vi "tabelUmrechnung.vi"(9 "Tabel Positon":dbl, 10 "Inspect":bool) -> (2 "In Range?":bool, 3 "Numerisch":dbl)   [LabVIEW 2020]
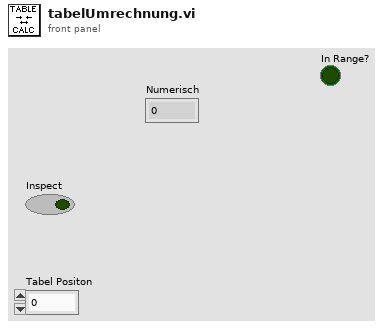
[diagram p1: front panel]
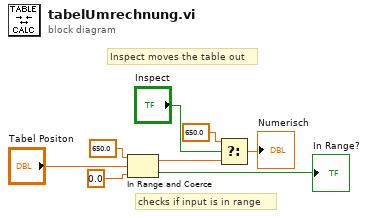
[diagram p0: block diagram]
diagram:
  # "checks if input is in range"
  # "Inspect moves the table out"
  n1 = In Range and Coerce(upper limit=650.0 ("Obergrenze"), x="Tabel Positon", lower limit=0.0) -> (coerced(x)=w4:dbl, In Range?=→"In Range?":bool)
  n2 = Select(t=650.0 ("Untergrenze"), s="Inspect", f=w4) -> (s? t:f=→"Numerisch":dbl)
